vi "Convert Endpoint to Endpoint String.vi"(11 "Endpoint":T1) -> (3 "Endpoint String":string)   [LabVIEW 2020, in "Routing and Faulting System Explorer.lvlib"]
uses:
  Routing and Faulting System Explorer.lvlib
  Shared/Alias Endpoint.ctl
  Shared/Routing and Faulting Shared.lvlib
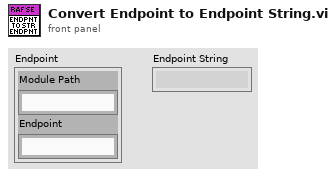
[diagram p1: front panel]
types:
  T1 = typedef "Routing and Faulting Shared.lvlib/Alias Endpoint.ctl" = cluster{"Module Path":string, "Endpoint":string}
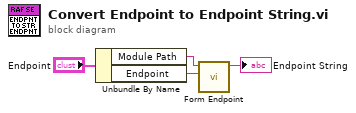
[diagram p0: block diagram]
diagram:
  n1 = Unbundle By Name("Endpoint") -> ("Module Path"=w2:string, "Endpoint"=w3:string)
  n2 = call "Form Endpoint.vi"("Endpoint"=w3, "Resource"=w2) -> ("Resource/Endpoint"=→"Endpoint String":string)  [unwired: 9 in]
